vi "Robot Global Data.vi"() -> ()   [LabVIEW 2020]
doc: "This global VI can contain as many global variables as you need. Place a control on the panel, give it a good name. To read or write to it from a VI, drag the icon to the diagram of that VI. You can also drag from the project. Click on the node to change which global you access. You shouldn't have multiple locations writing to a global or it will cause a race-condition."
uses:
  <vilib>/Rock Robotics/WPI/Camera/WPI_CameraImageSize.ctl
  <vilib>/Rock Robotics/WPI/DriverStation/WPI_DriverStationRobotMode2.ctl
  Drive Comands.ctl
  Direction Commands.ctl
panel:
  in  "Climber Rumble":bool
  in  "Wrong Color Left":bool
  in  "Wrong Color Right":bool
  in  "Align 90":bool
  out "Alliance Color":string
  in  "Auto Shot left":bool
  in  "Auto Shot Right":bool
  in  "Auto Intake":bool
  out "Right Color Match":string
  out "Left Color Match":string
  out "Auto Step":dbl
  out "Driver Axis":T1
  out "Driver Buttons":T2
  out "Auxillary Axis":T1
  out "Auxillary Buttons":T2
  in  "Reset Position":bool
  out "Front Left Drive Position":dbl
  in  "Gyro Adjustment":dbl
  in  "Auto Angle In":dbl
  in  "Zero Yaw":bool
  in  "Navx  Comp Yaw":dbl
  out "Driver POV":cluster{"POV":i16}
  out "Auxillary POV":cluster{"POV":i16}
  in  "Direction Commands":T3
  in  "Drive Commands":T4
  in  "Wheel Base Width":dbl=23.0
  in  "Wheel Base Length":dbl=20.0
  in  "Drive Speed Mode":string
  in  "Robot Mode":T5
  in  "image size":T6=enum."320x240"
  in  "Enable Vision":bool
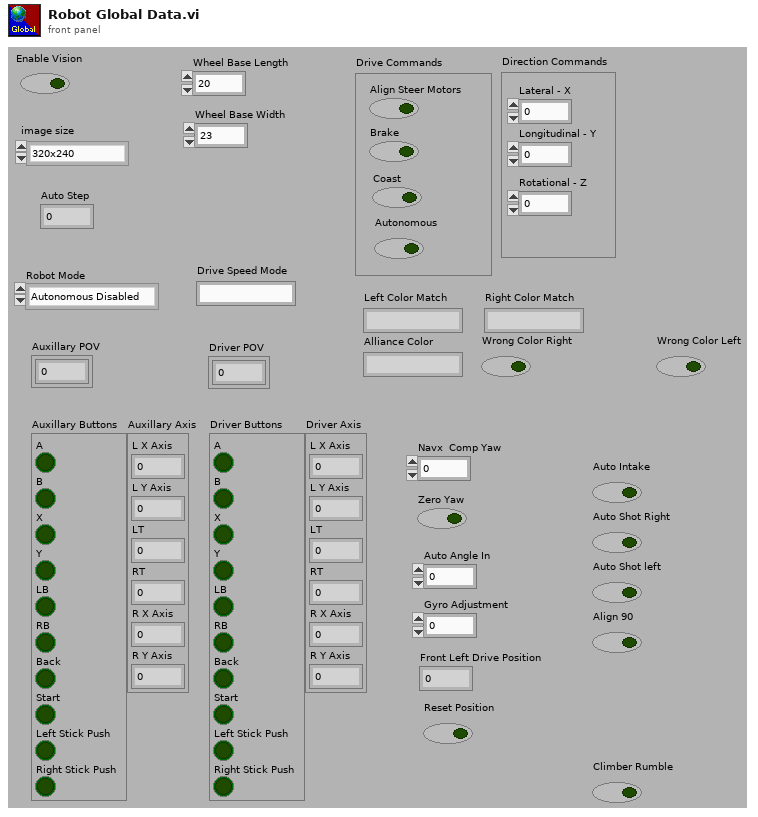
[diagram p1: front panel]
types:
  T1 = cluster{"L X Axis":dbl, "L Y Axis":dbl, "LT":dbl, "RT":dbl, "R X Axis":dbl, "R Y Axis":dbl}
  T2 = cluster{"A":bool, "B":bool, "X":bool, "Y":bool, "LB":bool, "RB":bool, "Back":bool, "Start":bool, "Left Stick Push":bool, "Right Stick Push":bool}
  T3 = typedef "Direction Commands.ctl" = cluster{"Lateral - X":dbl, "Longitudinal - Y":dbl, "Rotational - Z":dbl}
  T4 = typedef "Drive Comands.ctl" = cluster{"Align Steer Motors":bool, "Brake":bool, "Coast":bool, "Autonomous":bool}
  T5 = typedef "WPI_DriverStationRobotMode2.ctl" = enum16{"Autonomous Disabled", "Autonomous Enabled", "Teleop Disabled", "Teleop Enabled", "Disconnected", "Finish", "Test Disabled", "Test Enabled", "Emergency Stopped"}
  T6 = typedef "WPI_CameraImageSize.ctl" = enum16{"640x480", "320x240", "160x120", "Custom"}
diagram:
